vi "Write Vacuum Test Results.vi"(8 "error in (no error)":errorcluster, 10 "Fixture Name":string, 11 "Report Info":T1) -> (0 "error out":errorcluster, 3 "String":string)   [LabVIEW 2015]
uses:
  Controls/Report Config.ctl
  Tests/Controls/Test Results.ctl
  Tests/Controls/Step Result.ctl
  Tests/Controls/Test Information.ctl
  Tests/Controls/Vacuum Test.ctl
  Tests/Controls/Test Timing.ctl
  Tests/Controls/Vaccum Thresholds.ctl
  Tests/Controls/Helium Test.ctl
  Tests/Controls/Helium Thresholds.ctl
  <userlib>/_OpenG.lib/file/file.llb/Strip Path Extension - Path__ogtk.vi
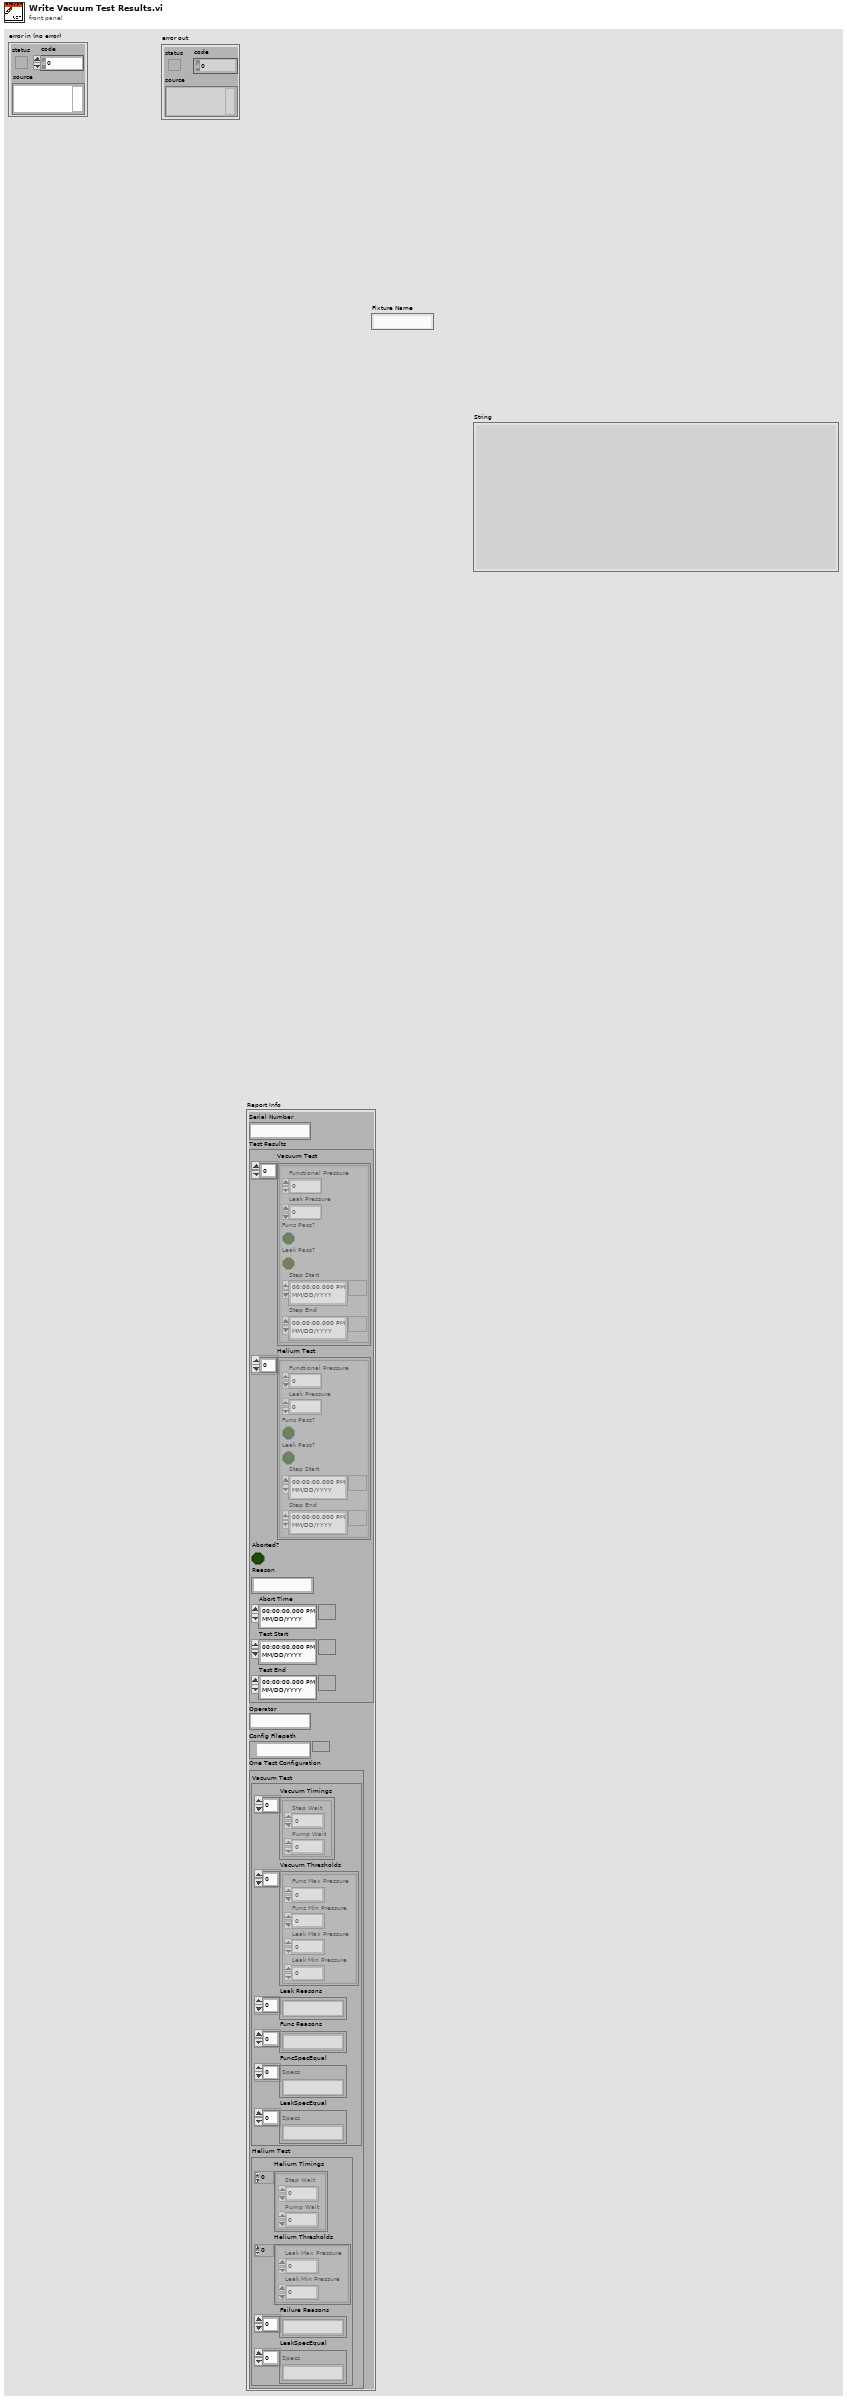
[diagram p1: front panel]
types:
  T1 = typedef "Report Config.ctl" = cluster{"Serial Number":string, "Test Results":T2, "Operator":string, "Config Filepath":path, "One Test Configuration":T4}
  T2 = typedef "Test Results.ctl" = cluster{"Vacuum Test":T3[], "Helium Test":T3[], "Aborted?":bool, "Reason":string, "Abort Time":timestamp, "Test Start":timestamp, "Test End":timestamp}
  T3 = typedef "Step Result.ctl" = cluster{"Functional Pressure":dbl, "Leak Pressure":dbl, "Func Pass?":bool, "Leak Pass?":bool, "Step Start":timestamp, "Step End":timestamp}
  T4 = typedef "Test Information.ctl" = cluster{"Vacuum Test":T5, "Helium Test":T8}
  T5 = typedef "Vacuum Test.ctl" = cluster{"Vacuum Timings":T6[], "Vacuum Thresholds":T7[], "Leak Reasons":string[], "Func Reasons":string[], "FuncSpecEqual":string[], "LeakSpecEqual":string[]}
  T6 = typedef "Test Timing.ctl" = cluster{"Step Wait":dbl, "Pump Wait":dbl}
  T7 = typedef "Vaccum Thresholds.ctl" = cluster{"Func Max Pressure":dbl, "Func Min Pressure":dbl, "Leak Max Pressure":dbl, "Leak Min Pressure":dbl}
  T8 = typedef "Helium Test.ctl" = cluster{"Helium Timings":T6[], "Helium Thresholds":T9[], "Failure Reasons":string[], "LeakSpecEqual":string[]}
  T9 = typedef "Helium Thresholds.ctl" = cluster{"Leak Max Pressure":dbl, "Leak Min Pressure":dbl}
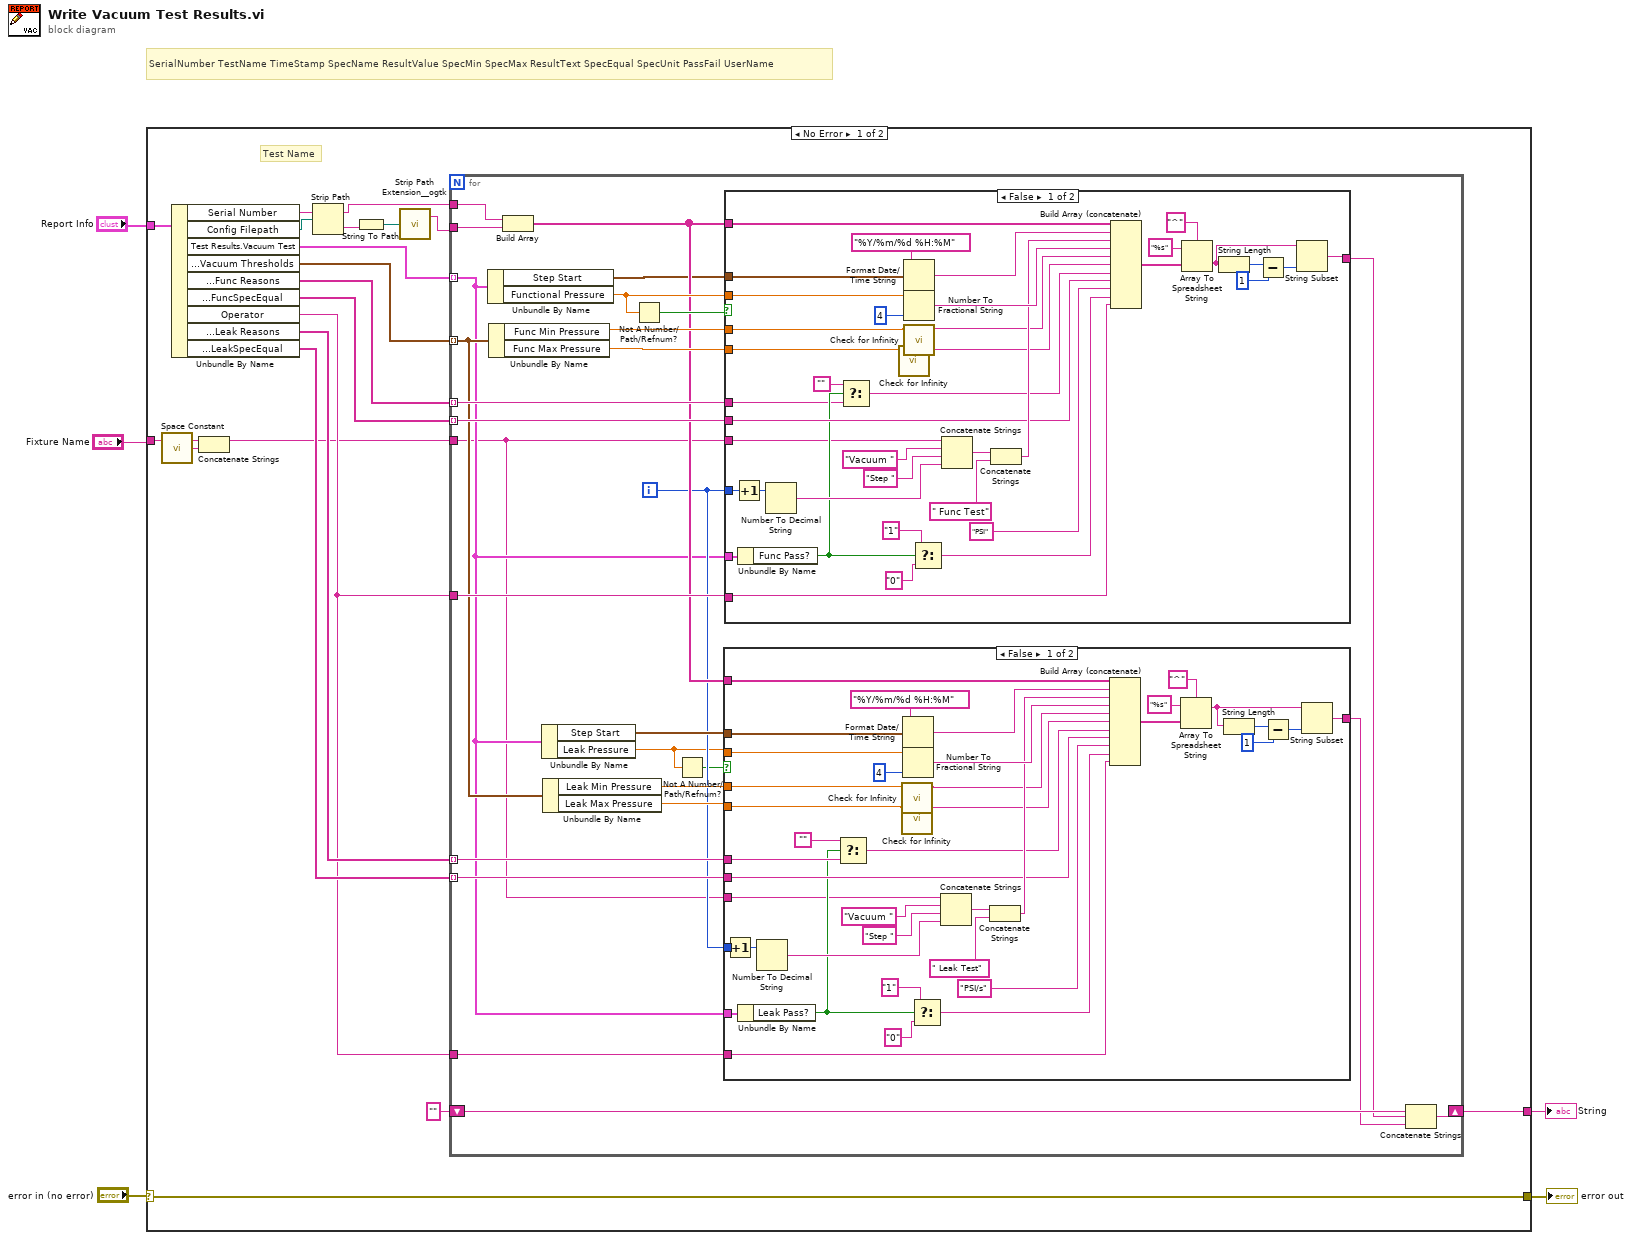
[diagram p0: block diagram]
diagram:
  # "SerialNumber\tTestName\tTimeStamp\tSpecName\tResultValue\tSpecMin\tSpecMax\tResultText\tSpecEqual\tSpecUnit\tPassFail\tUserName"
  n1 = case shown="No Error" "error in (no error)" {
    selector: "error in (no error)" -> [w10 w130]
    tunnel: [w10 w130] -> w3
    tunnel: "Report Info" -> [w24 _]
    tunnel: [w9 _] -> w2
    tunnel: "Fixture Name" -> [w8 _]
    frame No Error {
      # "Test Name"
      n2 = call <vilib>:"Space Constant.vi"() -> ("String"=w6:string)
      n3 = Unbundle By Name(w24) -> ("Serial Number"=w17:string, "Config Filepath"=w18:path, "Test Results.Vacuum Test"=w23:T3[], "One Test Configuration.Vacuum Test.Vacuum Thresholds"=w22:T7[], "One Test Configuration.Vacuum Test.Func Reasons"=w21:string[], "One Test Configuration.Vacuum Test.FuncSpecEqual"=w20:string[], "Operator"=w11:string, "One Test Configuration.Vacuum Test.Leak Reasons"=w13:string[], "One Test Configuration.Vacuum Test.LeakSpecEqual"=w12:string[])
      n4 = Concatenate Strings(w8, w6) -> (w7:string)
      n5 = Strip Path(path=w18) -> (name=w16:string)  [unwired: 1 out]
      n6 = String To Path(string=w16) -> (path=w14:path)
      n7 = call-poly <userlib>:"Strip Path Extension__ogtk.vi"("path"=w14) -> ("root"=w15:string)  [unwired: 1 out]
      n8 = for {
        tunnel: w23 -> [w30] mode=indexing
        tunnel: w22 -> [w36] mode=indexing
        tunnel: w21 -> [w49] mode=indexing
        tunnel: w20 -> [w48] mode=indexing
        tunnel: w11 -> [w47]
        tunnel: w17 -> [w46]
        shift-right: [w43] -> w9
        shift-left: "" -> [w42]
        tunnel: w15 -> [w40]
        tunnel: w13 -> [w33] mode=indexing
        tunnel: w12 -> [w32] mode=indexing
        tunnel: w11 -> [w27]
        tunnel: w7 -> [w25]
        i -> [w31]
        n9 = Unbundle By Name(w30) -> ("Step Start"=w38:timestamp, "Functional Pressure"=w45:dbl)
        n10 = Unbundle By Name(w36) -> ("Func Min Pressure"=w51:dbl, "Func Max Pressure"=w50:dbl)
        n11 = Build Array(w46, w40) -> (w39:string[])
        n12 = Unbundle By Name(w30) -> ("Step Start"=w37:timestamp, "Leak Pressure"=w29:dbl)
        n13 = Unbundle By Name(w36) -> ("Leak Min Pressure"=w35:dbl, "Leak Max Pressure"=w34:dbl)
        n14 = Not A Number/Path/Refnum?(number/path/refnum=w45) -> (NaN/Path/Refnum?=w44:bool)
        n15 = Not A Number/Path/Refnum?(number/path/refnum=w29) -> (NaN/Path/Refnum?=w28:bool)
        n16 = case shown="False" w28 {
          tunnel: w37 -> [w89 _]
          tunnel: w35 -> [w54 _]
          tunnel: w34 -> [w53 _]
          tunnel: w31 -> [w85 _]
          tunnel: w33 -> [w65 _]
          tunnel: w32 -> [w77 _]
          tunnel: w30 -> [w75 _]
          tunnel: w27 -> [w71 _]
          tunnel: w39 -> [w70 _]
          tunnel: w29 -> [w69 _]
          tunnel: [w57 _] -> w26
          tunnel: w25 -> [w56 _]
          frame False {
            n17 = Increment(x=w85) -> (x+1=w84:i32)
            n18 = Unbundle By Name(w75) -> ("Leak Pass?"=w64:bool)
            n19 = Number To Decimal String(number=w84) -> (decimal integer string=w81:string)  [unwired: 1 in]
            n20 = Select(t="", s=w64, f=w65) -> (s? t:f=w62:string)
            n21 = call "Check for Infinity.vi"("Number"=w54) -> ("F-format string"=w55:string)  [unwired: 10 in]
            n22 = call "Check for Infinity.vi"("Number"=w53) -> ("F-format string"=w52:string)  [unwired: 10 in]
            n23 = Format Date/Time String(time format string (%c)="%Y/%m/%d %H:%M", seconds (now)=w89) -> (date/time string=w87:string)  [unwired: 1 in]
            n24 = Number To Fractional String(number=w69, precision (6)=i16 4) -> (F-format string=w86:string)  [unwired: 2 in]
            n25 = Select(t="1" ("string"), s=w64, f="0" ("string")) -> (s? t:f=w72:string)
            n26 = Concatenate Strings(w56, "Vacuum " ("string"), "Step " ("string"), w81) -> (w80:string)
            n27 = Concatenate Strings(w80, " Leak Test" ("string")) -> (w78:string)
            n28 = Build Array (concatenate)(w70, w87, w78, w86, w55, w52, w62, w77, "PSI/s" ("string"), w72, w71) -> (w68:string[])
            n29 = Array To Spreadsheet String(delimiter (Tab)="^", array=w68, 3:"%s" ("format string")) -> (spreadsheet string=w58:string)
            n30 = String Length(string=w58) -> (length=w61:i32)
            n31 = Subtract(x=w61, y=1) -> (x-y=w59:i32)
            n32 = String Subset(string=w58, length (rest)=w59) -> (substring=w57:string)  [unwired: 1 in]
          }
          frame True {
          }
        }
        n33 = case shown="False" w44 {
          tunnel: w38 -> [w128 _]
          tunnel: w51 -> [w94 _]
          tunnel: w50 -> [w92 _]
          tunnel: w31 -> [w124 _]
          tunnel: w49 -> [w103 _]
          tunnel: w48 -> [w116 _]
          tunnel: w30 -> [w114 _]
          tunnel: w47 -> [w110 _]
          tunnel: w39 -> [w109 _]
          tunnel: w45 -> [w108 _]
          tunnel: [w96 _] -> w41
          tunnel: w25 -> [w95 _]
          frame False {
            n34 = Increment(x=w124) -> (x+1=w123:i32)
            n35 = Unbundle By Name(w114) -> ("Func Pass?"=w104:bool)
            n36 = Number To Decimal String(number=w123) -> (decimal integer string=w120:string)  [unwired: 1 in]
            n37 = Select(t="", s=w104, f=w103) -> (s? t:f=w101:string)
            n38 = call "Check for Infinity.vi"("Number"=w92) -> ("F-format string"=w91:string)  [unwired: 10 in]
            n39 = Format Date/Time String(time format string (%c)="%Y/%m/%d %H:%M", seconds (now)=w128) -> (date/time string=w126:string)  [unwired: 1 in]
            n40 = Number To Fractional String(number=w108, precision (6)=i16 4) -> (F-format string=w125:string)  [unwired: 2 in]
            n41 = call "Check for Infinity.vi"("Number"=w94) -> ("F-format string"=w93:string)  [unwired: 10 in]
            n42 = Select(t="1" ("string"), s=w104, f="0" ("string")) -> (s? t:f=w111:string)
            n43 = Concatenate Strings(w95, "Vacuum " ("string"), "Step " ("string"), w120) -> (w119:string)
            n44 = Concatenate Strings(w119, " Func Test" ("string")) -> (w117:string)
            n45 = Build Array (concatenate)(w109, w126, w117, w125, w93, w91, w101, w116, "PSI" ("string"), w111, w110) -> (w107:string[])
            n46 = Array To Spreadsheet String(delimiter (Tab)="^", array=w107, 3:"%s" ("format string")) -> (spreadsheet string=w97:string)
            n47 = String Length(string=w97) -> (length=w100:i32)
            n48 = Subtract(x=w100, y=1) -> (x-y=w98:i32)
            n49 = String Subset(string=w97, length (rest)=w98) -> (substring=w96:string)  [unwired: 1 in]
          }
          frame True {
          }
        }
        n50 = Concatenate Strings(w42, w41, w26) -> (w43:string)
      }
    }
    frame Error {
    }
  }
  "error out" <- w3
  "String" <- w2
